vi "handle_errors.vi"(0 "Exit Operation":bool, 5 "Restart Network":bool, 7 "Stop":bool, 9 "Halt":bool, 11 "error in (no error)":errorcluster) -> (15 "error out":errorcluster)   [LabVIEW 2013]
uses:
  <vilib>/Utility/error.llb/DialogType.ctl
  Globals.vi
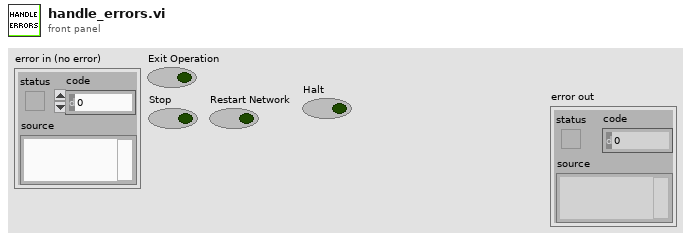
[diagram p1: front panel]
types:
  T1 = typedef "DialogType.ctl" = u16
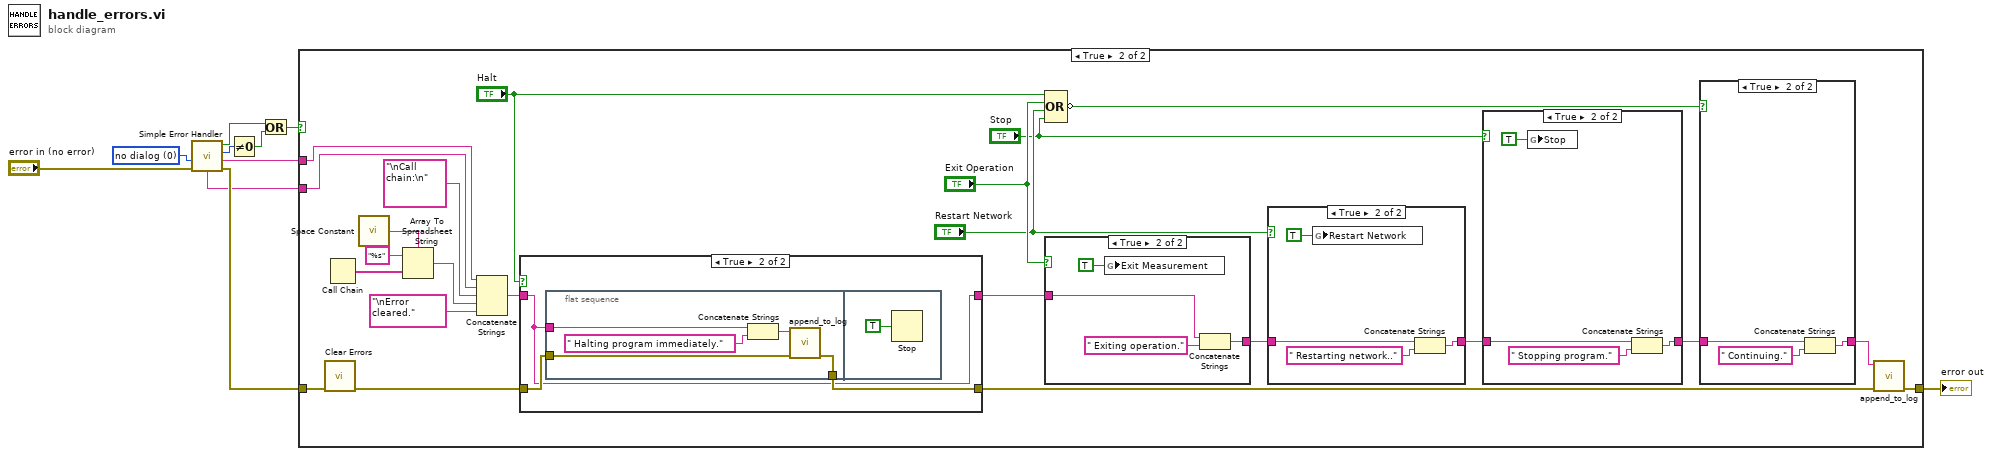
[diagram p0: block diagram]
diagram:
  w6 = T1 0 items=["no dialog", "OK message", "continue or stop message", "OK message + warnings", "continue/stop + warnings"] ("type of dialog (OK msg:1)")
  n1 = call <vilib>:"Simple Error Handler.vi"("type of dialog (OK msg:1)"=w6, "error in (no error)"="error in (no error)") -> ("error?"=w4:bool, "code out"=w3:i32, "source out"=w2:string, "error out"=w5:errorcluster, "message"=w1:string)  [unwired: 3 in]
  n2 = Not Equal To 0?(x=w3) -> (x != 0?=w10:bool)
  n3 = Or(x=w4, y=w10) -> (x .or. y?=w9:bool)
  n4 = case shown="True" w9 {
    tunnel: [w11 w34] -> w8
    tunnel: w5 -> [w11 w33]
    tunnel: w2 -> [_ w13]
    tunnel: w1 -> [_ w12]
    frame False {
    }
    frame True {
      n5 = call <vilib>:"Clear Errors.vi"("error in (no error)"=w33) -> ("error out"=w32:errorcluster)  [unwired: 6 in]
      n6 = Call Chain() -> (call chain=w16:string[])
      n7 = call <vilib>:"Space Constant.vi"() -> ("String"=w17:string)
      n8 = Array To Spreadsheet String(delimiter (Tab)=w17, array=w16, 3:"%s" ("format string")) -> (spreadsheet string=w18:string)
      n9 = Concatenate Strings(w13, w12, "\nCall chain:\n" ("string"), w18, "\nError cleared." ("F button name (\"Cancel\")")) -> (w14:string)
      n10 = case shown="True" "Halt" {
        tunnel: w14 -> [w39 w41]
        tunnel: w32 -> [w40 w43]
        tunnel: [w40 w42] -> w21
        tunnel: [w39 w41] -> w22
        frame False {
        }
        frame True {
          n11 = flat-sequence {
            tunnel: w41 -> [w48]
            tunnel: w43 -> [w46]
            tunnel: [w44] -> w42
            frame #0 {
              n12 = Concatenate Strings(w48, " Halting program immediately." ("string")) -> (w45:string)
              n13 = call "append_to_log.vi"("error in"=w46, "string"=w45) -> ("error out"=w44:errorcluster)  [unwired: 9 in]
            }
            frame #1 {
              n14 = Stop(stop? (T)=TRUE) -> ()
            }
          }
        }
      }
      n15 = Compound Arithmetic op=OR("Halt", "Exit Operation", "Restart Network", "Stop") -> (invert w25:bool)
      n16 = case shown="True" "Exit Operation" {
        tunnel: w22 -> [w60 w64]
        tunnel: [w60 w63] -> w31
        frame False {
        }
        frame True {
          n17 = global write "Globals.vi" "Exit Measurement"(TRUE ("Exit Measurement")) -> ()
          n18 = Concatenate Strings(w64, " Exiting operation." ("string")) -> (w63:string)
        }
      }
      n19 = case shown="True" "Restart Network" {
        tunnel: w31 -> [w50 w54]
        tunnel: [w50 w53] -> w30
        frame False {
        }
        frame True {
          n20 = global write "Globals.vi" "Restart Network"(TRUE ("Exit Measurement")) -> ()
          n21 = Concatenate Strings(w54, " Restarting network.." ("string")) -> (w53:string)
        }
      }
      n22 = case shown="True" "Stop" {
        tunnel: w30 -> [w55 w59]
        tunnel: [w55 w58] -> w24
        frame False {
        }
        frame True {
          n23 = global write "Globals.vi" "Stop"(TRUE ("Stop")) -> ()
          n24 = Concatenate Strings(w59, " Stopping program." ("string")) -> (w58:string)
        }
      }
      n25 = case shown="True" w25 {
        tunnel: w24 -> [w35 w38]
        tunnel: [w35 w36] -> w23
        frame False {
        }
        frame True {
          n26 = Concatenate Strings(w38, " Continuing." ("string")) -> (w36:string)
        }
      }
      n27 = call "append_to_log.vi"("error in"=w21, "string"=w23) -> ("error out"=w34:errorcluster)  [unwired: 9 in]
    }
  }
  "error out" <- w8
